vi "SEH Get Next Error.vi"() -> (0 "Transmission Error":errorcluster, 1 "Transmitted Error":errorcluster, 2 "Empty?":bool, 3 "Notification Info":T1)   [LabVIEW 2017]
doc: "Returns an error notification from the nofication queue. Notifications are enqueued using the Specific Error Handler."
uses:
  <userlib>/_SEH/Controls/Shared/SEH Notification Info.ctl
  <userlib>/_SEH/Controls/Shared/SEH Error Notification Command.ctl
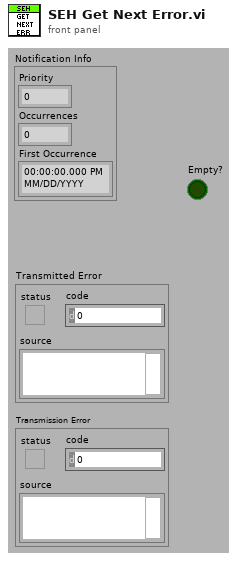
[diagram p1: front panel]
types:
  T1 = typedef "SEH Notification Info.ctl" = cluster{"Priority":i32, "Occurrences":i32, "First Occurrence":timestamp}
  T2 = typedef "SEH Error Notification Command.ctl" = enum16{"Init", "Send Error", "Check Error", "Invalid Command"}
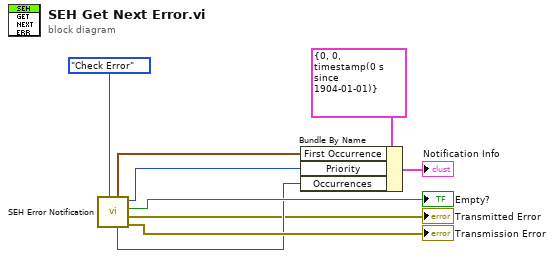
[diagram p0: block diagram]
diagram:
  n1 = call <userlib>:"SEH Error Notification.vi"("Command"=SEH_Error_Notification_Command."Check Error") -> ("Transmission Error"=→"Transmission Error":errorcluster, "Transmitted Error"=→"Transmitted Error":errorcluster, "Empty?"=→"Empty?":bool, "Priority Out"=w3:i32, "Occurrences"=w2:i32, "First Occurrence"=w4:timestamp)  [unwired: 5 in]
  n2 = Bundle By Name(cluster=T1 {"Priority"=0, "Occurrences"=0, "First Occurrence"=timestamp(0 s since 1904-01-01)} ("Notification Info"), "First Occurrence"=w4, "Priority"=w3, "Occurrences"=w2) -> (→"Notification Info":T1)
